vi "MacroAssert.vi"(8 "error in (no error)":errorcluster) -> (0 "error out":errorcluster)   [LabVIEW 2020, in "MacroAssert.lvlib"]
doc: "Presents an interface to create, edit, save, and execute user-defined macros."
uses:
  MacroAssert.lvlib
  Classes/Macro/Macro.lvclass
  Classes/Step/Step.lvclass
  <vilib>/Utility/miscctls.llb/LVRowAndColumnUnsignedTypeDef.ctl
  bd503c13-d10c-440e-ab5e-4e60baef5deb.vi
  SubVIs/FaKI State Machine/FaKI State Machine.lvlib
  CTLs/State Data.ctl
  CTLs/Hotkey Values.ctl
  CTLs/FGV Actions.ctl
  CTLs/Hotkey Type.ctl
  CTLs/Refs.ctl
  fa5aba67-e91f-4216-ac5c-c17457851557.vi
  CTLs/Report Data.ctl
  CTLs/Edit Action.ctl
  <vilib>/Utility/miscctls.llb/LVPositionTypeDef.ctl
  <vilib>/Utility/inputDevices.llb/closeKeyboard.vi
panel:
  in  "Report Path":path
  out "Status":string
  in  "Add Step 2":bool
  in  "Dbl Click":T1
  in  "Macro Steps":i32(listbox)
  out "Abort Hotkey":string
  out "Metadata":string
  in  "Description":string
  out "Resolutions":cluster{"Width":i16, "Height":i16}[](array[cluster])
  out "n Monitors":i32
  out "Macro Hotkey":string
  in  "Start/Stop":bool
  in  "N":i32 caption="Times to Repeat\n(-1 = indefinitely)" min=-1
  in  "Activation Type":enum32{"Hotkey", "Automatic"}(radio)
  out "Row":i32
  in  "Clear Steps":bool
  in  "Delete Step":bool
  in  "Insert Step":bool
  in  "Add Step":bool
  in  "Modify Step":bool
  in  "Macro Name":string(combo)
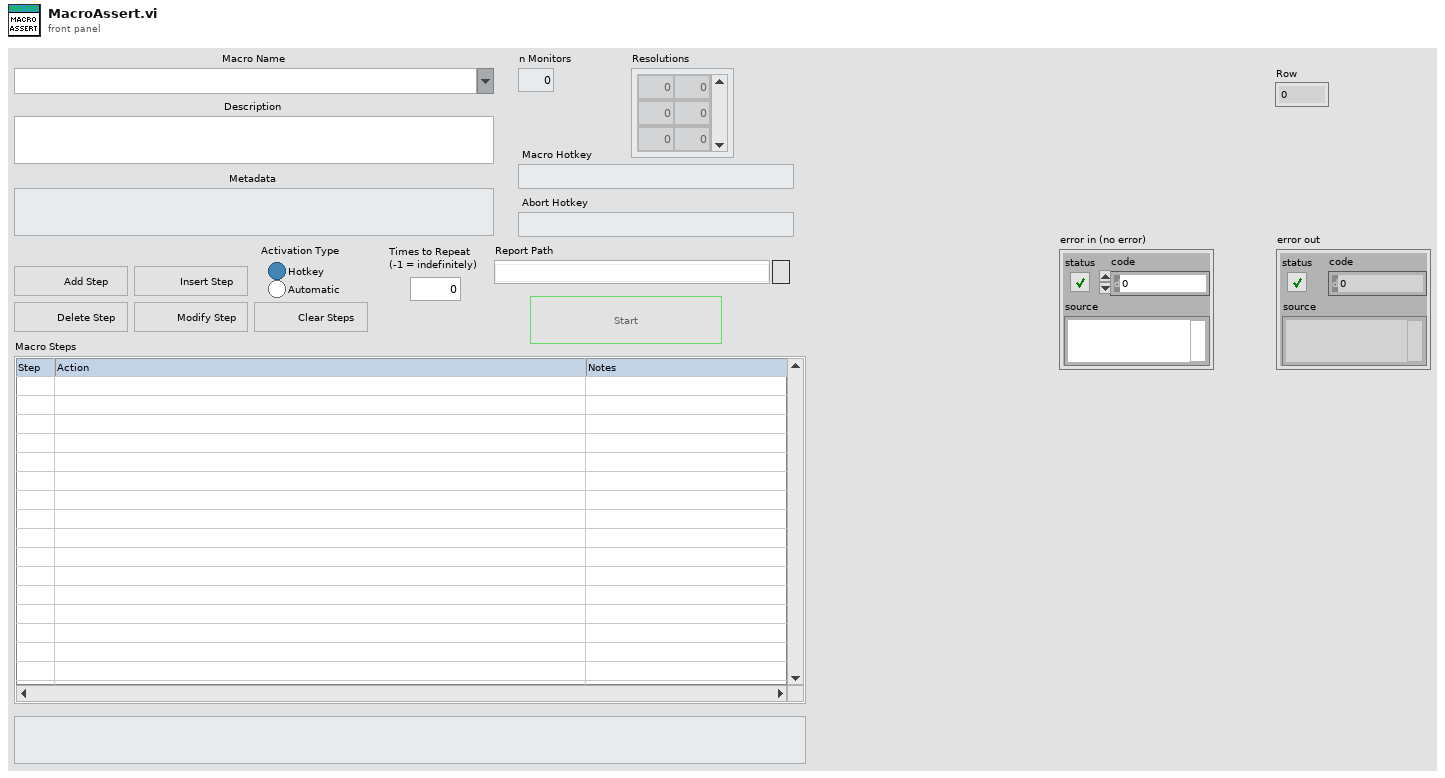
[diagram p1: front panel]
types:
  T1 = cluster{"Insert Before":bool, "Insert After":bool, "Modify Step 2":bool, "Delete Step 2":bool}
  T2 = typedef "LVPoint32TypeDef.ctl" = cluster{"Horizontal":i32, "Vertical":i32}
  T3 = enum32{"Invalid", "Standard", "Closed", "Hidden", "Minimized", "Maximized"}
  T4 = enum32{"invalid app kind", "Development System", "Run Time System", "Student Edition", "Embedded LabVIEW", "Evaluation", "Custom"}
  T5 = typedef "MacroAssert.lvlib/State Data.ctl" = cluster{"Core":cluster{"Current VI Reference":refnum<vi>, "Close Panel on Exit?":bool}, "Macro":cluster{"New":refnum<class "Macro.lvclass">, "Saved":refnum<class "Macro.lvclass">}, "Step":i32, "n":i32, "Hotkey Values":T6, "Keyboard":refnum<k1>, "Macro Active?":bool, "Macro Names":string[], "Rcount":i32, "Refs":T7, "Resolutions":cluster{"Width":i16, "Height":i16}[], "App Data Dir":path, "Start Time":timestamp, "Report Data":T8[]}
  T6 = typedef "MacroAssert.lvlib/Hotkey Values.ctl" = cluster{"Macro Hotkey":enum16{"0", "1", "2", "3", "4", "5", "6", "7", "8", "9", "A", "B", "C", "D", "E", "F", "G", "H", "I", "J", "K", "L", "M", "N", "O", "P", "Q", "R", "S", "T", "U", "V", "W", "X", "Y", "Z", "F1", "F2", "F3", "F4", "F5", "F6", "F7", "F8", "F9", "F10", "F11", "F12", "F13", "F14", "F15", "ADD", "BACK", "BACKSLASH", "CAPITAL", "COMMA", "DECIMAL", "DELETE", "DIVIDE", "DOWN", "END", "EQUALS", "ESCAPE", "GRAVE (`)", "HOME", "INSERT", "LBRACKET", "LCONTROL", "LEFT", "L ALT", "LSHIFT", "LWIN", "MINUS", "MULTIPLY", "NEXT", "NUMLOCK", "NUMPAD_0", "NUMPAD_1", "NUMPAD_2", "NUMPAD_3", "NUMPAD_4", "NUMPAD_5", "NUMPAD_6", "NUMPAD_7", "NUMPAD_8", "NUMPAD_9", "PAUSE", "PERIOD", "PRIOR (PG UP)", "RBRACKET", "RCONTROL", "RETURN", "RIGHT", "R ALT", "RSHIFT", "RWIN", "SCROLL", "SEMICOLON", "SLASH", "SPACE", "SUBTRACT", "TAB", "UP", "ENTER (num pad)", "' (quote)"}[], "Abort Hotkey":enum16{"0", "1", "2", "3", "4", "5", "6", "7", "8", "9", "A", "B", "C", "D", "E", "F", "G", "H", "I", "J", "K", "L", "M", "N", "O", "P", "Q", "R", "S", "T", "U", "V", "W", "X", "Y", "Z", "F1", "F2", "F3", "F4", "F5", "F6", "F7", "F8", "F9", "F10", "F11", "F12", "F13", "F14", "F15", "ADD", "BACK", "BACKSLASH", "CAPITAL", "COMMA", "DECIMAL", "DELETE", "DIVIDE", "DOWN", "END", "EQUALS", "ESCAPE", "GRAVE (`)", "HOME", "INSERT", "LBRACKET", "LCONTROL", "LEFT", "L ALT", "LSHIFT", "LWIN", "MINUS", "MULTIPLY", "NEXT", "NUMLOCK", "NUMPAD_0", "NUMPAD_1", "NUMPAD_2", "NUMPAD_3", "NUMPAD_4", "NUMPAD_5", "NUMPAD_6", "NUMPAD_7", "NUMPAD_8", "NUMPAD_9", "PAUSE", "PERIOD", "PRIOR (PG UP)", "RBRACKET", "RCONTROL", "RETURN", "RIGHT", "R ALT", "RSHIFT", "RWIN", "SCROLL", "SEMICOLON", "SLASH", "SPACE", "SUBTRACT", "TAB", "UP", "ENTER (num pad)", "' (quote)"}[]}
  T7 = typedef "MacroAssert.lvlib/Refs.ctl" = cluster{"Name":refnum<vi>, "Description":refnum<vi>, "Start":refnum<vi>, "Steps":refnum<vi>, "Simple Refs":refnum<vi>[]}
  T8 = typedef "MacroAssert.lvlib/Report Data.ctl" = cluster{"Step":string, "Pass?":bool, "Actual Value":variant}
  T9 = typedef "MacroAssert.lvlib/Edit Action.ctl" = enum16{"Add", "Insert", "Modify", "Delete", "Insert Before", "Insert After", "Modify 2", "Delete 2", "Clear All"}
  T10 = typedef "LVRowAndColumnUnsignedTypeDef.ctl" = cluster{"Row":u32, "Column":u32}
  T11 = enum8{"Enabled", "Disabled", "Disabled and Grayed Out"}
  T12 = typedef "LVPositionTypeDef.ctl" = cluster{"Left":i32, "Top":i32}
  T13 = typedef "MacroAssert.lvlib/Hotkey Type.ctl" = enum16{"Macro Hotkey", "Abort Hotkey"}
  T14 = typedef "MacroAssert.lvlib/FGV Actions.ctl" = enum16{"Read", "Write"}
  T15 = enum16{"0", "1", "2", "3", "4", "5", "6", "7", "8", "9", "A", "B", "C", "D", "E", "F", "G", "H", "I", "J", "K", "L", "M", "N", "O", "P", "Q", "R", "S", "T", "U", "V", "W", "X", "Y", "Z", "F1", "F2", "F3", "F4", "F5", "F6", "F7", "F8", "F9", "F10", "F11", "F12", "F13", "F14", "F15", "ADD", "BACK", "BACKSLASH", "CAPITAL", "COMMA", "DECIMAL", "DELETE", "DIVIDE", "DOWN", "END", "EQUALS", "ESCAPE", "GRAVE (`)", "HOME", "INSERT", "LBRACKET", "LCONTROL", "LEFT", "L ALT", "LSHIFT", "LWIN", "MINUS", "MULTIPLY", "NEXT", "NUMLOCK", "NUMPAD_0", "NUMPAD_1", "NUMPAD_2", "NUMPAD_3", "NUMPAD_4", "NUMPAD_5", "NUMPAD_6", "NUMPAD_7", "NUMPAD_8", "NUMPAD_9", "PAUSE", "PERIOD", "PRIOR (PG UP)", "RBRACKET", "RCONTROL", "RETURN", "RIGHT", "R ALT", "RSHIFT", "RWIN", "SCROLL", "SEMICOLON", "SLASH", "SPACE", "SUBTRACT", "TAB", "UP", "ENTER (num pad)", "' (quote)"}[]
  T16 = typedef "LVAllMonitorsDisplayTypeDef.ctl" = cluster{"Bounds":cluster{"Left":i16, "Top":i16, "Right":i16, "Bottom":i16}, "Depth":i16}[]
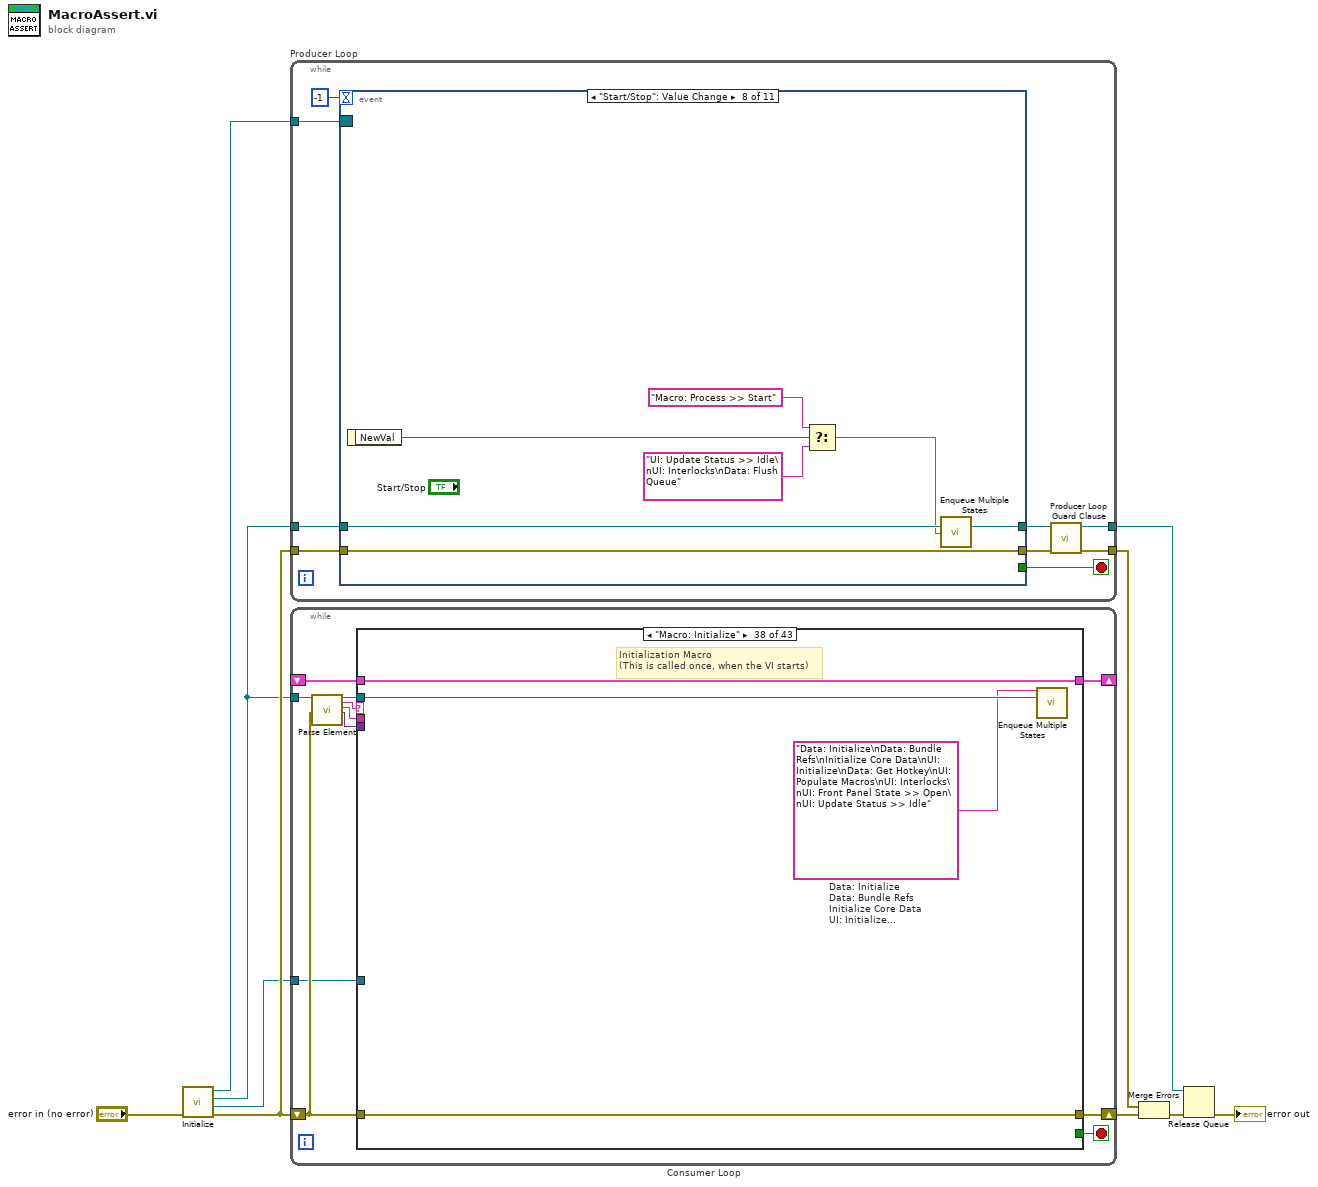
[diagram p0: block diagram]
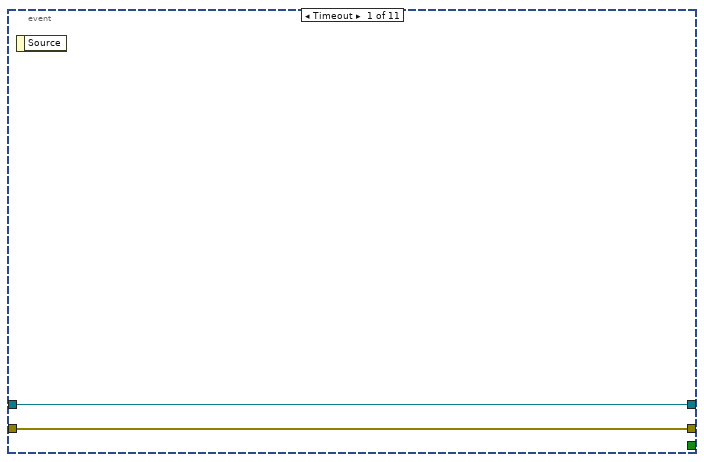
[diagram p2: hidden frame]
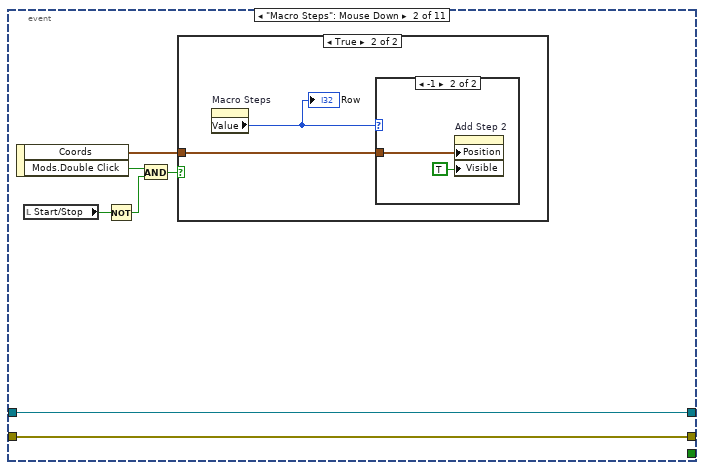
[diagram p3: hidden frame]
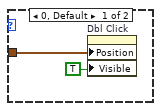
[diagram p5: hidden frame]
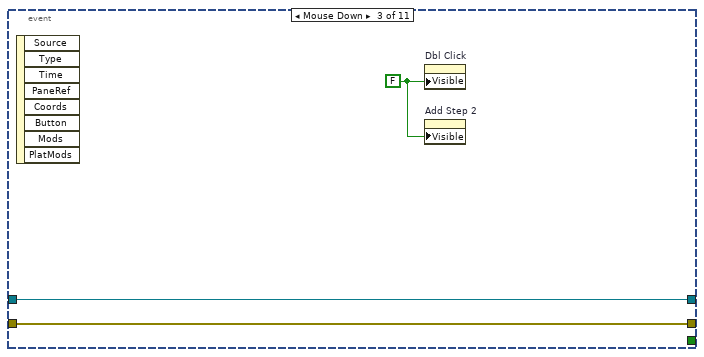
[diagram p6: hidden frame]
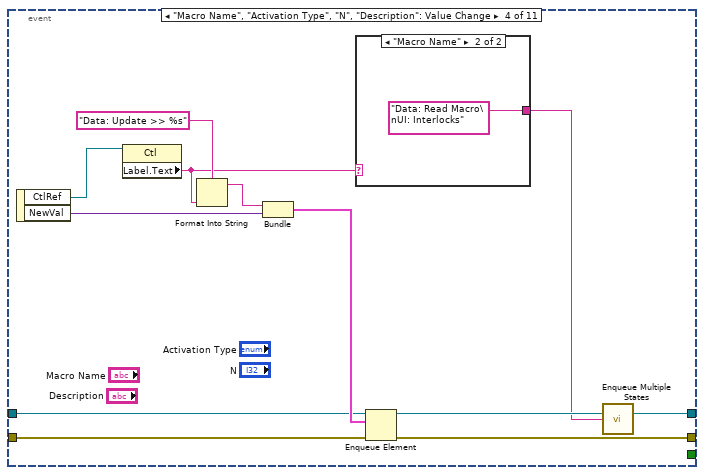
[diagram p7: hidden frame]
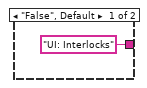
[diagram p8: hidden frame]
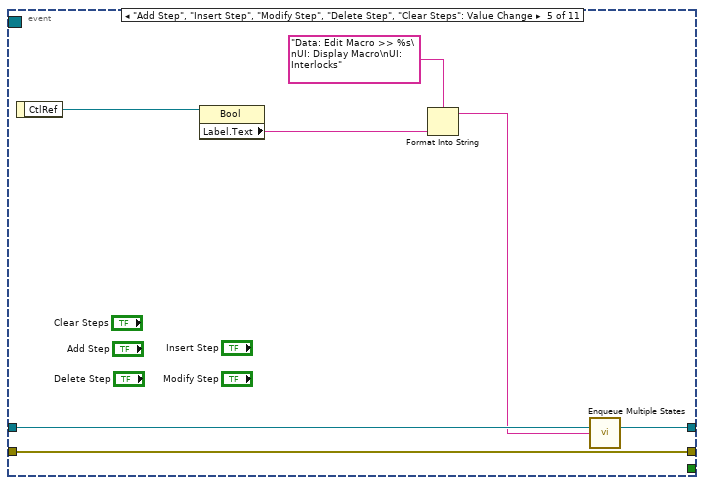
[diagram p9: hidden frame]
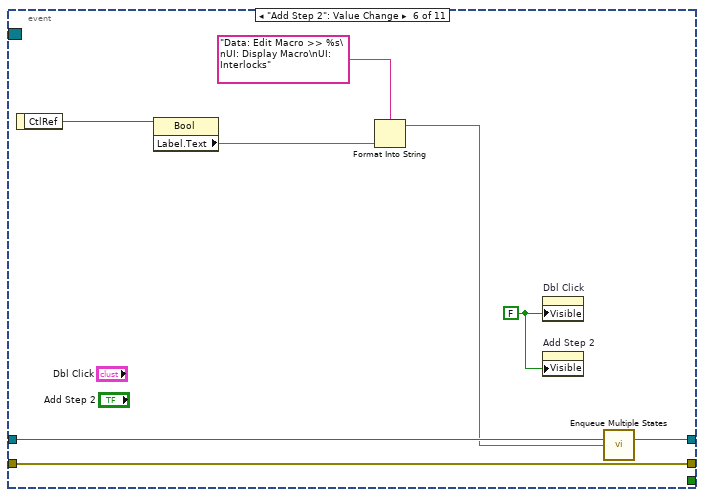
[diagram p10: hidden frame]
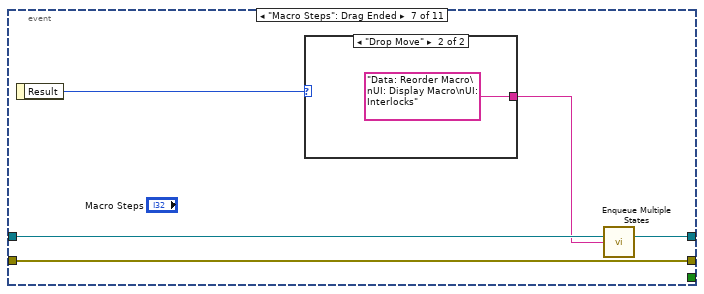
[diagram p11: hidden frame]
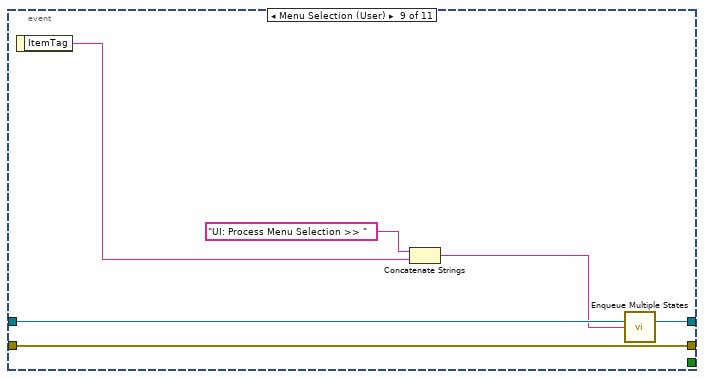
[diagram p13: hidden frame]
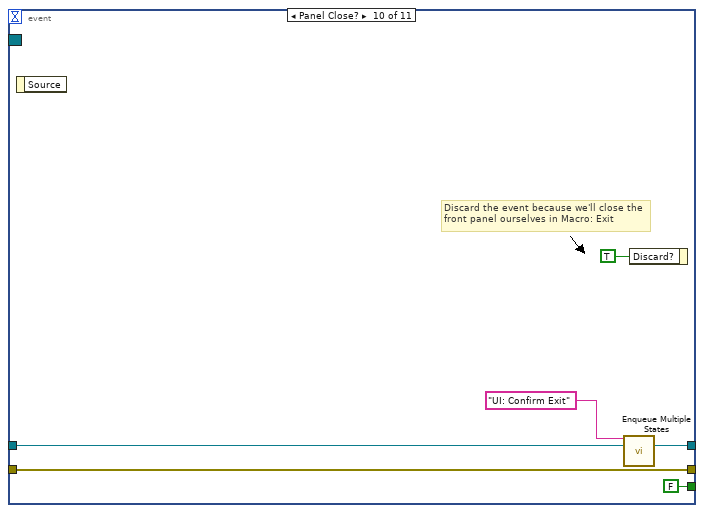
[diagram p14: hidden frame]
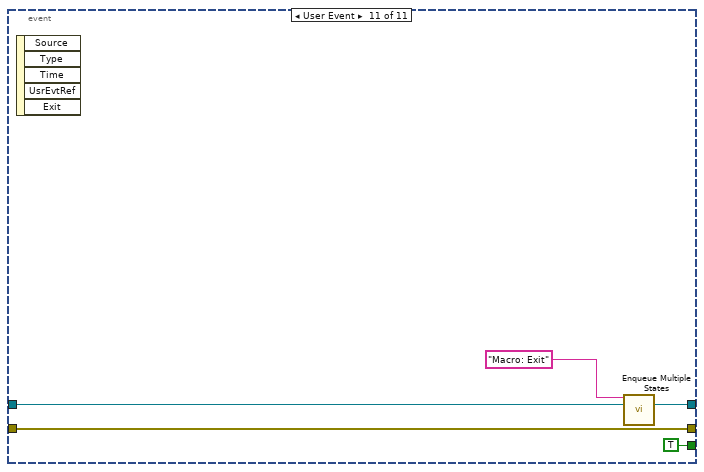
[diagram p15: hidden frame]
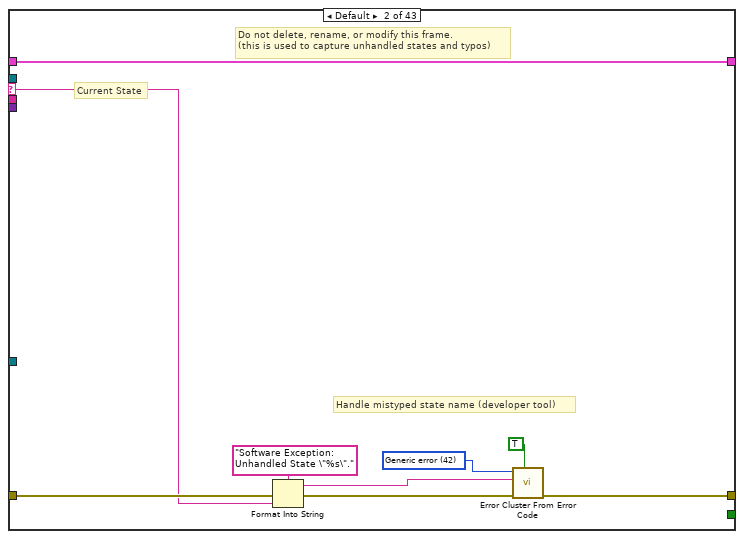
[diagram p17: hidden frame]
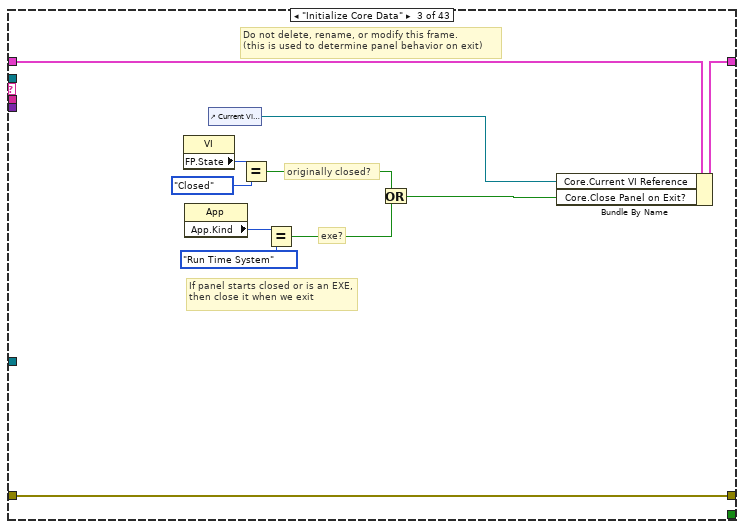
[diagram p18: hidden frame]
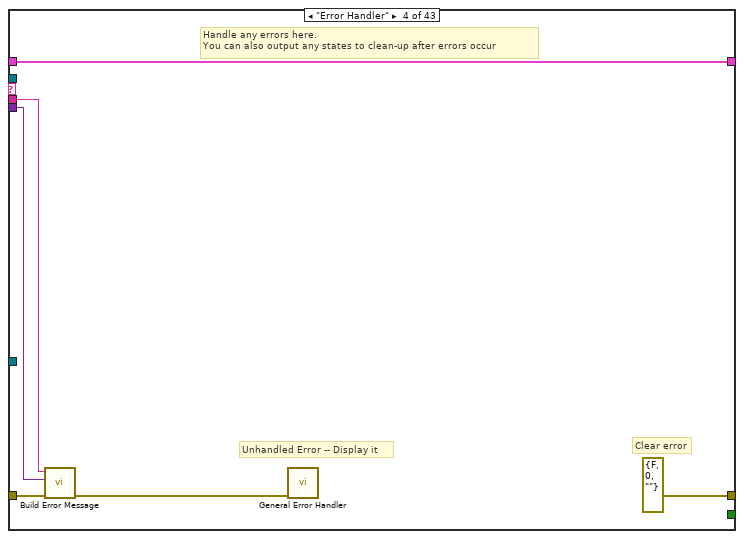
[diagram p19: hidden frame]
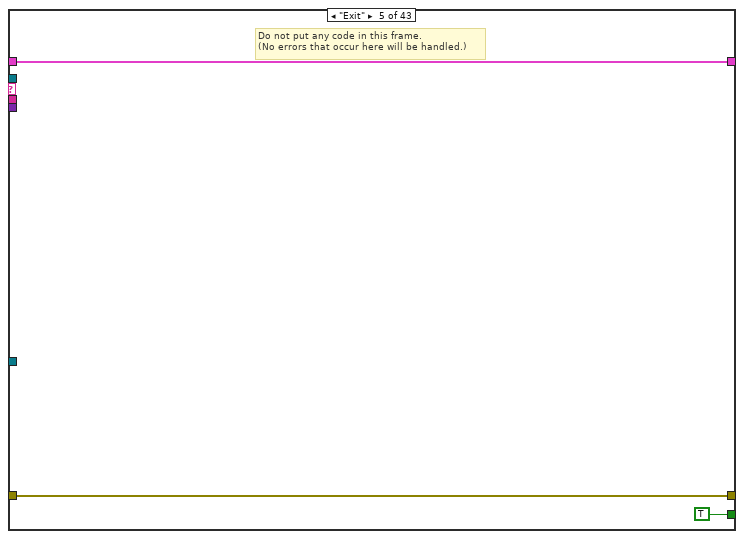
[diagram p20: hidden frame]
diagram:
  n1 = call "Initialize.vi"("error in (no error)"="error in (no error)") -> ("error out"=w5:errorcluster, "Exit Event"=w3:refnum<user-event>, "Queue"=w2:refnum<queue>, "Event Registration Refnum"=w1:refnum<event-registration>)  [unwired: 7 in]
  n2 = while "Producer Loop" {
    tunnel: w1 -> [w13]
    tunnel: w2 -> [w15]
    tunnel: [w18] -> w10
    tunnel: w5 -> [w17]
    tunnel: [w19] -> w8
    stop <- w12 stop-if-true
    n3 = event shown="[7] \"Start/Stop\": Value Change" {
      selector: w13 -> [_ _ _ _ _ _ _ _ _ _ _]
      dyn-events: _ -> [_ _ _ _ _ _ _ _ _ _ _]
      timeout: -1 ("Timeout") -> [_ _ _ _ _ _ _ _ _ _ _]
      tunnel: [w21 w28 w37 w45 w58 w66 w71 w79 w85 w91 w96] -> w16
      tunnel: w17 -> [w21 w28 w37 w48 w58 w66 w71 w79 w85 w91 w96]
      tunnel: w15 -> [w20 w26 w36 w38 w56 w63 w70 w75 w84 w88 w94]
      tunnel: [w20 w26 w36 w47 w55 w62 w69 w76 w83 w87 w93] -> w14
      tunnel: [_ _ _ _ _ _ _ _ _ FALSE TRUE] -> w12
      event Timeout {
        n4 = event-data() -> ()  [unwired: 1 in, 1 out]
      }
      event "Macro Steps": Mouse Down {
        n5 = event-data() -> ("Coords"=w27:T2, "Mods.Double Click"=w23:bool)  [unwired: 1 in]
        n6 = local read "Start/Stop"() -> (w25:bool)
        n7 = Not(x=w25) -> (.not. x?=w24:bool)
        n8 = And(x=w23, y=w24) -> (x .and. y?=w22:bool)
        n9 = case shown="True" w22 {
          tunnel: w27 -> [_ w30]
          frame False {
          }
          frame True {
            n10 = property on="Macro Steps" class="MCListbox (strict)"() -> ("Value"=w29:i32)  [unwired: 2 in, 2 out]
            "Row" <- w29
            n11 = case shown="-1" w29 {
              tunnel: w30 -> [w31 w33]
              frame 0, Default {
                n12 = property on="Dbl Click" class="Clust"("Position"=w31, "Visible"=TRUE) -> ()  [unwired: 2 in, 2 out]
              }
              frame -1 {
                n13 = property on="Add Step 2" class="Bool"("Position"=w33, "Visible"=TRUE) -> ()  [unwired: 2 in, 2 out]
              }
            }
          }
        }
      }
      event Mouse Down {
        w35 = FALSE ("Visible")
        n14 = event-data() -> ()  [unwired: 1 in, 8 out]
        n15 = property on="Dbl Click" class="Clust"("Visible"=w35) -> ()  [unwired: 2 in, 2 out]
        n16 = property on="Add Step 2" class="Bool"("Visible"=w35) -> ()  [unwired: 2 in, 2 out]
      }
      event "Macro Name", "Activation Type", "N", "Description": Value Change {
        n17 = event-data() -> ("CtlRef"=w44:refnum<vi>, "NewVal"=w41:variant)  [unwired: 1 in]
        n18 = property class="Ctl"(reference=w44) -> ("Label.Text"=w40:string)  [unwired: 1 in, 2 out]
        n19 = Format Into String(format string="Data: Update >> %s", w40) -> (resulting string=w42:string)  [unwired: 2 in, 1 out]
        n20 = Bundle(w42, "NewVal"=w41) -> (w39:cluster{string, "NewVal":variant})  [unwired: 1 in]
        n21 = case shown="\"Macro Name\"" w40 {
          tunnel: ["UI: Interlocks" ("string") "Data: Read Macro\nUI: Interlocks" ("string")] -> w46
          frame "False", Default {
          }
          frame "Macro Name" {
          }
        }
        n22 = Enqueue Element(queue=w38, element=w39, error in (no error)=w48) -> (queue out=w49:refnum<queue>, error out=w45:errorcluster)  [unwired: 1 in, 1 out]
        n23 = call "Enqueue Multiple States.vi"("queue in"=w49, "State(s) at Back"=w46) -> ("queue out"=w47:refnum<queue>)  [unwired: 13 in]
      }
      event "Add Step", "Insert Step", "Modify Step", "Delete Step", "Clear Steps": Value Change {
        n24 = event-data() -> ("CtlRef"=w57:refnum<vi>)  [unwired: 1 in]
        n25 = property class="Bool"(reference=w57) -> ("Label.Text"=w54:string)  [unwired: 1 in, 2 out]
        n26 = Format Into String(format string="Data: Edit Macro >> %s\nUI: Display Macro\nUI: Interlocks", w54) -> (resulting string=w52:string)  [unwired: 2 in, 1 out]
        n27 = call "Enqueue Multiple States.vi"("queue in"=w56, "State(s) at Back"=w52) -> ("queue out"=w55:refnum<queue>)  [unwired: 13 in]
      }
      event "Dbl Click.Insert Before", "Dbl Click.Insert After", "Dbl Click.Modify Step 2", "Dbl Click.Delete Step 2", "Add Step 2": Value Change {
        w64 = FALSE ("Visible")
        n28 = event-data() -> ("CtlRef"=w65:refnum<vi>)  [unwired: 1 in]
        n29 = property class="Bool"(reference=w65) -> ("Label.Text"=w60:string)  [unwired: 1 in, 2 out]
        n30 = Format Into String(format string="Data: Edit Macro >> %s\nUI: Display Macro\nUI: Interlocks", w60) -> (resulting string=w59:string)  [unwired: 2 in, 1 out]
        n31 = property on="Dbl Click" class="Clust"("Visible"=w64) -> ()  [unwired: 2 in, 2 out]
        n32 = property on="Add Step 2" class="Bool"("Visible"=w64) -> ()  [unwired: 2 in, 2 out]
        n33 = call "Enqueue Multiple States.vi"("queue in"=w63, "State(s) at Back"=w59) -> ("queue out"=w62:refnum<queue>)  [unwired: 13 in]
      }
      event "Macro Steps": Drag Ended {
        n34 = event-data() -> ("Result"=w67:enum16{"Drop Cancel", "Drop Move", "Drop Copy"})  [unwired: 1 in]
        n35 = case shown="\"Drop Move\"" w67 {
          tunnel: [_ "Data: Reorder Macro\nUI: Display Macro\nUI: Interlocks" ("State(s) at Back")] -> w68
          frame "Drop Cancel", Default {
          }
          frame "Drop Move" {
          }
        }
        n36 = call "Enqueue Multiple States.vi"("queue in"=w70, "State(s) at Back"=w68) -> ("queue out"=w69:refnum<queue>)  [unwired: 13 in]
      }
      event "Start/Stop": Value Change {
        n37 = event-data() -> ("NewVal"=w78:bool)  [unwired: 1 in]
        n38 = Select(t="Macro: Process >> Start", s=w78, f="UI: Update Status >> Idle\nUI: Interlocks\nData: Flush Queue") -> (s? t:f=w74:string)
        n39 = call "Enqueue Multiple States.vi"("queue in"=w75, "State(s) at Back"=w74) -> ("queue out"=w76:refnum<queue>)  [unwired: 13 in]
      }
      event Menu Selection (User) {
        n40 = event-data() -> ("ItemTag"=w81:string)  [unwired: 1 in]
        n41 = Concatenate Strings("UI: Process Menu Selection >> ", w81) -> (w80:string)
        n42 = call "Enqueue Multiple States.vi"("queue in"=w84, "State(s) at Back"=w80) -> ("queue out"=w83:refnum<queue>)  [unwired: 13 in]
      }
      event Panel Close? {
        # "Discard the event because we'll close the front panel ourselves in Macro: Exit"
        n43 = event-data() -> ()  [unwired: 1 in, 1 out]
        n44 = call "Enqueue Multiple States.vi"("State(s) at Front"="UI: Confirm Exit", "queue in"=w88) -> ("queue out"=w87:refnum<queue>)  [unwired: 13 in]
        n45 = event-data("Discard?"=TRUE) -> ()  [unwired: 1 in, 1 out]
      }
      event User Event {
        n46 = event-data() -> ()  [unwired: 1 in, 5 out]
        n47 = call "Enqueue Multiple States.vi"("State(s) at Front"="Macro: Exit", "queue in"=w94) -> ("queue out"=w93:refnum<queue>)  [unwired: 13 in]
      }
    }
    n48 = call "Producer Loop Guard Clause.vi"("error in (no error)"=w16, "queue in"=w14) -> ("error out"=w19:errorcluster, "queue out"=w18:refnum<queue>)  [unwired: 8 in]
  }
  n49 = while "Consumer Loop" {
    shift-right: [w98] -> _
    shift-left: _ -> [w103]
    shift-right: [w105] -> w7
    shift-left: w5 -> [w106]
    tunnel: w2 -> [w107]
    tunnel: w3 -> [w97]
    stop <- w104 stop-if-true
    n50 = call "Parse Element.vi"("queue in"=w107, "error in (no error)"=w106) -> ("queue out"=w102:refnum<queue>, "State"=w101:string, "Arg"=w100:string, "Data"=w99:variant)  [unwired: 14 in]
    n51 = case shown="\"Macro: Initialize\"" w101 {
      selector: w101 -> [_ w110 _ _ _ _ _ _ _ _ _ _ _ _ _ _ _ _ _ _ _ _ _ _ _ _ _ _ _ _ _ _ _ _ _ _ _ _ _ _ _ _ _]
      tunnel: w102 -> [_ _ _ _ _ _ _ _ _ _ _ _ _ _ _ _ w337 w358 _ _ _ _ _ _ _ w478 _ _ _ w547 w562 _ _ w583 w592 _ _ w627 w631 w632 w709 _ w725]
      tunnel: w100 -> [_ _ _ w131 _ _ _ _ w168 _ _ _ w253 _ _ _ _ _ _ _ _ _ w393 w401 _ w479 _ _ w501 _ _ _ _ _ _ _ _ _ _ w636 _ _ _]
      tunnel: w103 -> [w108 w112 w124 w134 w138 w139 _ w154 w169 w223 w237 w243 w254 w303 w315 w327 w333 w359 w367 w368 w372 w390 w396 w403 w475 w483 w487 w499 w502 w546 w565 w573 w576 w582 w593 w616 w622 w625 w629 w633 w713 w715 w724]
      tunnel: [w109 w114 w128 errorcluster {"status"=FALSE, "code"=0, "source"=""} ("error out") w137 w140 w142 w155 w164 w224 w235 w244 w256 w304 w320 w328 w335 w360 w365 w369 w375 w391 w394 w404 w476 w481 w489 w497 w503 w540 w561 w571 w574 w580 w589 w610 w623 w626 w630 w637 w714 w716 w721] -> w105
      tunnel: w106 -> [w109 w113 w128 w133 w137 w140 w147 w155 w167 w224 w229 w245 w256 w304 w320 w329 w336 w360 w364 w369 w375 w391 w395 w405 w476 w482 w490 w497 w503 w549 w566 w572 w575 w580 w589 w614 w623 w626 w630 w637 w714 w716 w722]
      tunnel: [_ _ _ _ TRUE _ _ _ _ _ _ _ _ _ _ _ _ _ _ _ _ _ _ _ _ _ _ _ _ _ _ _ _ _ _ _ _ _ _ _ _ _ _] -> w104
      tunnel: w99 -> [_ _ _ w130 _ _ _ _ w166 _ _ _ _ _ _ _ _ _ _ _ _ _ _ _ _ _ _ _ _ _ _ _ _ _ _ _ _ _ _ _ _ _ _]
      tunnel: [w108 w112 w129 w134 w138 w139 w143 w153 w165 w222 w236 w243 w255 w302 w314 w326 w334 w359 w367 w368 w370 w390 w396 w403 w475 w483 w488 w499 w502 w546 w565 w573 w576 w582 w591 w616 w622 w625 w629 w635 w713 w715 w723] -> w98
      tunnel: w97 -> [_ _ _ _ _ _ _ _ _ _ _ _ _ _ _ _ _ _ _ _ _ _ _ _ _ _ _ _ _ _ _ _ _ _ _ w608 _ _ _ _ _ _ _]
      frame "---------- Core ----------" {
        # "Do not put any code in this frame.\n(it is a separator no-op)"
      }
      frame Default {
        w117 = 42 items=["No error", "Argument error", "Memory is full", "Out of zone", "End of file", "File already open", "Generic file I/O error", "File not found", "File permission error", "Disk is full", "Duplicate path", "Too many files open", "System feature not enabled", "Resource file not found", "Cannot add resource", "Resource not found", "Image not found", "Image memory error", "Pen does not exist", "Config type invalid", "Config token not found", "Config parse error", "Config memory error", "Bad external code format", "Bad external code offset", "External code not present", "Null window", "Destroy window error", "Null menu", "Print aborted", "Bad print record", "Print driver error", "Windows error during printing", "Memory error during printing", "Print dialog error", "Generic print error", "Invalid device refnum", "Device not found", "Device parameter error", "Device unit error", "Cannot open device", "Device call aborted", "Generic error", "Cancelled by user", "Object ID too low", "Object ID too high", "Object not in heap", "Unknown heap", "Unknown object (invalid DefProc)", "Unknown object (DefProc not in table)", "Message out of range", "Invalid (null) method", "Unknown message", "Manager call not supported", "Bad address", "Network operation in progress", "Network operation timed out", "Connection is busy", "Network attribute not supported", "Network error", "Address in use", "System out of memory", "Connection aborted", "Connection refused", "Not connected", "Already connected", "Connection closed", "Initialization error (interapplication manager)", "Bad occurrence", "Wait on unbound occurrence handler", "Occurrence queue overflow", "Datalog type conflict", "Unused", "Unrecognized type (interapplication manager)", "Memory corrupt", "Failed to make temporary DLL", "Old CIN version", "Drag socket not found", "Failed to load drop-object", "Failed to register OLE object", "Failed to release OLE object", "Format specifier type mismatch", "Unknown format specifier", "Too few format specifiers", "Too many format specifiers", "Scan failed", "Newer CIN version", "Error converting to variant", "Runtime menu error", "Password tampered", "Variant attribute not found", "Incompatible variant data type", "Event data is not available", "Event Store is not present", "Occurrence is not found", "Event Queue is not created", "Event info is not available", "Refnum passed is NULL", "Error retrieving Class GUID", "Error retrieving CoClass GUID", "Error retrieving TypeLib GUID.", "Bad built application magic bytes.", "Specific driver is different from the specific driver associated with the Logical Name.", "There is no session opened to the class driver.", "Max Error", "MAX - Error with config objects", "MAX - Error loading configuration", "MAX - Group not supported"]
        # "Current State"
        # "Do not delete, rename, or modify this frame.\n(this is used to capture unhandled states and typos)"
        # "Handle mistyped state name (developer tool)"
        n52 = Format Into String(format string="Software Exception: Unhandled State \"%s\"." ("message"), error in=w113, w110) -> (resulting string=w116:string, error out=w115:errorcluster)  [unwired: 1 in]
        n53 = call <vilib>:"Error Cluster From Error Code.vi"("show call chain? (False)"=TRUE, "error in (no error)"=w115, "error message (\"\")"=w116, "error code (0)"=w117) -> ("error out"=w114:errorcluster)  [unwired: 5 in]
      }
      frame "Initialize Core Data" {
        # "Do not delete, rename, or modify this frame.\n(this is used to determine panel behavior on exit)"
        # "originally closed?"
        # "exe?"
        # "If panel starts closed or is an EXE, then close it when we exit"
        n54 = property class="VI"() -> ("FP.State"=w121:T3)  [unwired: 2 in, 2 out]
        n55 = property class="App"() -> ("App.Kind"=w127:T4)  [unwired: 2 in, 2 out]
        n56 = control-ref of="Current VI Reference"() -> (w122:refnum<vi>)
        n57 = Equal?(x=w121, y=T3."Closed" ("Front Panel Window:State")) -> (x = y?=w119:bool)
        n58 = Equal?(x=w127, y=T4."Run Time System" ("Application:Kind")) -> (x = y?=w125:bool)
        n59 = Or(x=w119, y=w125) -> (x .or. y?=w123:bool)
        n60 = Bundle By Name(cluster=w124, "Core.Current VI Reference"=w122, "Core.Close Panel on Exit?"=w123) -> (w129:T5)
      }
      frame "Error Handler" {
        # "Unhandled Error -- Display it"
        # "Handle any errors here.\nYou can also output any states to clean-up after errors occur"
        # "Clear error"
        n61 = call "Build Error Message.vi"("error in (no error)"=w133, "Data"=w130, "Arg"=w131) -> ("error out"=w132:errorcluster)  [unwired: 8 in]
        n62 = call <vilib>:"General Error Handler.vi"("error in (no error)"=w132) -> ()  [unwired: 10 in, 5 out]
      }
      frame "Exit" {
        # "Do not put any code in this frame.\n(No errors that occur here will be handled.)"
      }
      frame "---------- Data ----------" {
        # "Do not put any code in this frame.\n(It is a separator no-op. You can make a copy of this frame to create a new Data frame)"
      }
      frame "Data: Initialize" {
        # "Initialize the shift-register data, here."
        n63 = call <vilib>:"Intialize Keyboard.vi"("error in (no error)"=w147) -> ("error out"=w146:errorcluster, "device ID"=w144:refnum<k1>)  [unwired: 9 in]
        n64 = call "App Data Directory.vi"("error in (no error)"=w146) -> ("error out"=w142:errorcluster, "App Data Directory"=w141:path)  [unwired: 9 in]
        n65 = Bundle By Name(cluster=T5 {"Core"={"Current VI Reference"=refnum, "Close Panel on Exit?"=FALSE}, "Macro"={"New"=refnum, "Saved"=refnum}, "Step"=0, "n"=0, "Hotkey Values"={"Macro Hotkey"=[], "Abort Hotkey"=[]}, "Keyboard"=refnum, "Macro Active?"=FALSE, "Macro Names"=[], "Rcount"=0, "Refs"={"Name"=refnum, "Description"=refnum, "Start"=refnum, "Steps"=refnum, "Simple Refs"=[]}, "Resolutions"=[], "App Data Dir"=path "", "Start Time"=timestamp(0 s since 1904-01-01), "Report Data"=[]}, "Keyboard"=w144, "App Data Dir"=w141) -> (w143:T5)
      }
      frame "Data: Bundle Refs" {
        n66 = control-ref of="Activation Type"() -> (w158:refnum<vi>)
        n67 = control-ref of="Macro Name"() -> (w156:refnum<vi>)
        n68 = control-ref of="Add Step"() -> (w163:refnum<vi>)
        n69 = control-ref of="Delete Step"() -> (w161:refnum<vi>)
        n70 = control-ref of="Insert Step"() -> (w160:refnum<vi>)
        n71 = control-ref of="Modify Step"() -> (w162:refnum<vi>)
        n72 = control-ref of="Clear Steps"() -> (w159:refnum<vi>)
        n73 = control-ref of="N"() -> (w157:refnum<vi>)
        n74 = control-ref of="Macro Steps"() -> (w148:refnum<vi>)
        n75 = control-ref of="Macro Name"() -> (w152:refnum<vi>)
        n76 = control-ref of="Start/Stop"() -> (w150:refnum<vi>)
        n77 = control-ref of="Description"() -> (w151:refnum<vi>)
        n78 = Build Array(w163, w161, w160, w162, w159, w158, w157, w156) -> (w149:refnum<vi>[])
        n79 = Bundle By Name(cluster=w154, "Refs.Name"=w152, "Refs.Description"=w151, "Refs.Start"=w150, "Refs.Steps"=w148, "Refs.Simple Refs"=w149) -> (w153:T5)
      }
      frame "Data: Update" {
        n80 = case shown="\"Macro Name\"" w168 {
          selector: w168 -> [w170 _ _ _ _ _]
          tunnel: w169 -> [w173 w177 w187 w197 w206 w218]
          tunnel: w167 -> [w174 w181 w191 w201 w211 w221]
          tunnel: w166 -> [_ w180 w190 w200 w210 w220]
          tunnel: [w173 w176 w186 w196 w207 w217] -> w165
          tunnel: [w172 w178 w189 w199 w209 w216] -> w164
          frame Default {
            n81 = call "Unhandled String Argument--error.vi"("Argument"=w170) -> ("error out"=w171:errorcluster)  [unwired: 10 in]
            n82 = Merge Errors(w174, w171) -> (w172:errorcluster)
          }
          frame "Macro Name" {
            n83 = Variant To Data(error in=w181, type="", Variant=w180) -> (data=w175:string, error out=w178:errorcluster)
            n84 = in-place {
              in-place-border: w175 -> [w182]
              n85 = in-place-cluster #1(w177) -> ("Macro.New"=w184:refnum<class "Macro.lvclass">)
              n86 = property class="Macro.lvclass"(reference=w184, "Accessors:Name"=w182) -> (reference out=w183:refnum<class "Macro.lvclass">)  [unwired: 1 in, 1 out]
              n87 = in-place-cluster #1("Macro.New"=w183) -> (w176:T5)
            }
          }
          frame "Activation Type" {
            n88 = Variant To Data(error in=w191, type=enum32{"Hotkey", "Automatic"}."Hotkey" ("FP CTLs.Type"), Variant=w190) -> (data=w185:enum32{"Hotkey", "Automatic"}, error out=w189:errorcluster)
            n89 = in-place {
              in-place-border: w185 -> [w192]
              n90 = in-place-cluster #2(w187) -> ("Macro.New"=w194:refnum<class "Macro.lvclass">)
              n91 = property class="Macro.lvclass"(reference=w194, "Accessors:Activation Type"=w192) -> (reference out=w193:refnum<class "Macro.lvclass">)  [unwired: 1 in, 1 out]
              n92 = in-place-cluster #2("Macro.New"=w193) -> (w186:T5)
            }
          }
          frame "N" {
            n93 = Variant To Data(error in=w201, type=0 ("FP CTLs.N"), Variant=w200) -> (data=w195:i32, error out=w199:errorcluster)
            n94 = in-place {
              in-place-border: w195 -> [w202]
              n95 = in-place-cluster #3(w197) -> ("Macro.New"=w204:refnum<class "Macro.lvclass">)
              n96 = property class="Macro.lvclass"(reference=w204, "Accessors:N"=w202) -> (reference out=w203:refnum<class "Macro.lvclass">)  [unwired: 1 in, 1 out]
              n97 = in-place-cluster #3("Macro.New"=w203) -> (w196:T5)
            }
          }
          frame "Description" {
            n98 = Variant To Data(error in=w211, type="" ("FP CTLs.N"), Variant=w210) -> (data=w205:string, error out=w209:errorcluster)
            n99 = in-place {
              in-place-border: w205 -> [w212]
              n100 = in-place-cluster #4(w206) -> ("Macro.New"=w214:refnum<class "Macro.lvclass">)
              n101 = property class="Macro.lvclass"(reference=w214, "Accessors:Description"=w212) -> (reference out=w213:refnum<class "Macro.lvclass">)  [unwired: 1 in, 1 out]
              n102 = in-place-cluster #4("Macro.New"=w213) -> (w207:T5)
            }
          }
          frame "Macro Active?" {
            n103 = Variant To Data(error in=w221, type=FALSE, Variant=w220) -> (data=w219:bool, error out=w216:errorcluster)
            n104 = Bundle By Name(cluster=w218, "Macro Active?"=w219) -> (w217:T5)
          }
        }
      }
      frame "Data: Increment Step" {
        n105 = in-place {
          n106 = in-place-cluster #5(w223) -> ("Step"=w226:i32)
          n107 = Increment(x=w226) -> (x+1=w225:i32)
          n108 = in-place-cluster #5("Step"=w225) -> (w222:T5)
        }
      }
      frame "Data: Get Hotkey" {
        n109 = call "App Config INI.vi"("error in (no error)"=w229) -> ("error out"=w228:errorcluster, "App Config"=w227:path)  [unwired: 9 in]
        n110 = call "Get Hotkey.vi"("error in (no error)"=w228, "File Path"=w227) -> ("error out"=w235:errorcluster, "Hotkey Values"=w233:T6)  [unwired: 8 in]
        n111 = Unbundle By Name(w233) -> ("Macro Hotkey"=w232:T15, "Abort Hotkey"=w230:T15)
        n112 = Bundle By Name(cluster=w237, "Hotkey Values"=w233) -> (w236:T5)
        n113 = call "Convert Hotkey to String.vi"("Hotkey"=w232) -> ("String"=→"Macro Hotkey":string)  [unwired: 10 in]
        n114 = call "Convert Hotkey to String.vi"("Hotkey"=w230) -> ("String"=→"Abort Hotkey":string)  [unwired: 10 in]
      }
      frame "Data: Build Report" {
        n115 = Unbundle By Name(w243) -> ("Macro.New"=w242:refnum<class "Macro.lvclass">, "Report Data"=w241:T8[])
        n116 = Empty String/Path?(string/path="Report Path") -> (empty?=w239:bool)
        n117 = Not(x=w239) -> (.not. x?=w238:bool)
        n118 = case shown="True" w238 {
          tunnel: w245 -> [w246 w251]
          tunnel: [w246 w250] -> w244
          tunnel: w242 -> [_ w249]
          tunnel: w241 -> [_ w248]
          tunnel: "Report Path" -> [_ w247]
          frame False {
          }
          frame True {
            n119 = call-dynamic "Build Report.vi"("error in (no error)"=w251, "Report Data"=w248, "Path"=w247, "Macro in"=w249) -> ("error out"=w250:errorcluster)  [unwired: 6 in, 1 out]
          }
        }
      }
      frame "Data: Edit Macro" {
        n120 = local read "Row"() -> (w252:i32)
        n121 = in-place {
          in-place-border: w253 -> [w258]
          in-place-border: w252 -> [w257]
          n122 = in-place-cluster #6(w254) -> ("Macro.New"=w260:refnum<class "Macro.lvclass">)
          n123 = case shown="\"Add Step\"" w258 {
            tunnel: w260 -> [w261 w263 w266 w269 w272 w276 w278 w282 w287 w291 w295]
            tunnel: [w261 w262 w265 w268 w271 w275 w277 w281 w286 w290 w294] -> w259
            tunnel: w257 -> [_ _ _ _ _ _ w279 w284 w288 w292 _]
            frame Default {
            }
            frame "Add Step" {
              n124 = call-dynamic "Edit.vi"("Action"=Edit_Action."Add", "Macro in"=w263) -> ("Macro out"=w262:refnum<class "Macro.lvclass">)  [unwired: 8 in, 1 out]
            }
            frame "Insert Step" {
              n125 = call-dynamic "Edit.vi"("Action"=Edit_Action."Insert", "Macro in"=w266) -> ("Macro out"=w265:refnum<class "Macro.lvclass">)  [unwired: 8 in, 1 out]
            }
            frame "Modify Step" {
              n126 = call-dynamic "Edit.vi"("Action"=Edit_Action."Modify", "Macro in"=w269) -> ("Macro out"=w268:refnum<class "Macro.lvclass">)  [unwired: 8 in, 1 out]
            }
            frame "Delete Step" {
              n127 = call-dynamic "Edit.vi"("Action"=Edit_Action."Delete", "Macro in"=w272) -> ("Macro out"=w271:refnum<class "Macro.lvclass">)  [unwired: 8 in, 1 out]
            }
            frame "Add Step 2" {
              n128 = call-dynamic "Edit.vi"("Action"=Edit_Action."Add", "Macro in"=w276) -> ("Macro out"=w275:refnum<class "Macro.lvclass">)  [unwired: 8 in, 1 out]
            }
            frame "Insert Before" {
              n129 = call-dynamic "Edit.vi"("Action"=Edit_Action."Insert Before", "Step"=w279, "Macro in"=w278) -> ("Macro out"=w277:refnum<class "Macro.lvclass">)  [unwired: 7 in, 1 out]
            }
            frame "Insert After" {
              n130 = Increment(x=w284) -> (x+1=w283:i32)
              n131 = call-dynamic "Edit.vi"("Action"=Edit_Action."Insert After", "Step"=w283, "Macro in"=w282) -> ("Macro out"=w281:refnum<class "Macro.lvclass">)  [unwired: 7 in, 1 out]
            }
            frame "Modify Step 2" {
              n132 = call-dynamic "Edit.vi"("Action"=Edit_Action."Modify 2", "Step"=w288, "Macro in"=w287) -> ("Macro out"=w286:refnum<class "Macro.lvclass">)  [unwired: 7 in, 1 out]
            }
            frame "Delete Step 2" {
              n133 = call-dynamic "Edit.vi"("Action"=Edit_Action."Delete 2", "Step"=w292, "Macro in"=w291) -> ("Macro out"=w290:refnum<class "Macro.lvclass">)  [unwired: 7 in, 1 out]
            }
            frame "Clear Steps" {
              n134 = call "Confirm Clear"() -> ("OK"=w296:bool)  [unwired: 10 in, 1 out]
              n135 = case shown="True" w296 {
                tunnel: w295 -> [w297 w300]
                tunnel: [w297 w299] -> w294
                frame False {
                }
                frame True {
                  n136 = property on="Macro Steps" class="MCListbox (strict)"("TopLeft"=T10 {"Row"=0, "Column"=0} ("Index Values")) -> ()  [unwired: 2 in, 2 out]
                  n137 = call-dynamic "Edit.vi"("Action"=Edit_Action."Clear All", "Macro in"=w300) -> ("Macro out"=w299:refnum<class "Macro.lvclass">)  [unwired: 8 in, 1 out]
                }
              }
            }
          }
          n138 = in-place-cluster #6("Macro.New"=w259) -> (w255:T5)
        }
      }
      frame "Data: Bundle Macro" {
        n139 = in-place {
          n140 = in-place-cluster #7(w303) -> ("Resolutions"=w309:cluster{"Width":i16, "Height":i16}[], "Macro.New"=w312:refnum<class "Macro.lvclass">)
          n141 = property class="Macro.lvclass"(reference=w312) -> (reference out=w310:refnum<class "Macro.lvclass">, "Accessors:Date Created"=w307:timestamp)  [unwired: 1 in, 1 out]
          n142 = Get Date/Time In Seconds() -> (seconds since 1Jan1904=w305:timestamp)
          n143 = Not Equal To 0?(x=w307) -> (x != 0?=w308:bool)
          n144 = Select(t=w307, s=w308, f=w305) -> (s? t:f=w306:timestamp)
          n145 = property class="Macro.lvclass"(reference=w310, "Accessors:Resolutions"=w309, "Accessors:Date Created"=w306, "Accessors:Date Updated"=w305) -> (reference out=w311:refnum<class "Macro.lvclass">)  [unwired: 1 in, 1 out]
          n146 = in-place-cluster #7("Resolutions"=w309, "Macro.New"=w311) -> (w302:T5)
        }
      }
      frame "Data: Reorder Macro" {
        n147 = property on="Macro Steps" class="MCListbox (strict)"() -> ("ItemNames"=w319:string[][])  [unwired: 2 in, 2 out]
        n148 = Index Array(array=w319, index (col)=0 ("disabled index (col)")) -> (element=w317:string[])  [unwired: 1 in]
        n149 = Decimal String To Number(string=w317) -> (number=w316:i32[])  [unwired: 2 in, 1 out]
        n150 = Decrement(x=w316) -> (x-1=w313:i32[])
        n151 = in-place {
          in-place-border: w313 -> [w321]
          n152 = in-place-cluster #8(w315) -> ("Macro.New"=w323:refnum<class "Macro.lvclass">)
          n153 = call-dynamic "Reorder Steps.vi"("New Order"=w321, "Macro in"=w323) -> ("Macro out"=w322:refnum<class "Macro.lvclass">)  [unwired: 8 in, 1 out]
          n154 = in-place-cluster #8("Macro.New"=w322) -> (w314:T5)
        }
      }
      frame "Data: Save Macro" {
        n155 = Unbundle By Name(w327) -> ("Macro.New"=w324:refnum<class "Macro.lvclass">)
        n156 = call-dynamic "Write to File.vi"("error in (no error)"=w329, "Macro in"=w324) -> ("error out"=w328:errorcluster, "Macro out"=w325:refnum<class "Macro.lvclass">)  [unwired: 8 in]
        n157 = Bundle By Name(cluster=w327, "Macro.New"=w325, "Macro.Saved"=w325) -> (w326:T5)
      }
      frame "Data: Read Macro" {
        n158 = Unbundle By Name(w333) -> ("Macro Names"=w330:string[], "App Data Dir"=w331:path)
        n159 = in-place {
          in-place-border: w336 -> [w348]
          in-place-border: [w347] -> w335
          in-place-border: w331 -> [w343]
          in-place-border: w330 -> [w341]
          n160 = in-place-cluster #9(w333) -> ("Macro.New"=w346:refnum<class "Macro.lvclass">)  [unwired: 1 out]
          n161 = property class="Macro.lvclass"(reference=w346) -> (reference out=w342:refnum<class "Macro.lvclass">, "Accessors:Name"=w339:string)  [unwired: 1 in, 1 out]
          n162 = Search 1D Array(1D array=w341, element=w339) -> (index of element=w340:i32)  [unwired: 1 in]
          n163 = case shown="0, Default" w340 {
            tunnel: w348 -> [w354 w357]
            tunnel: [w353 w357] -> w347
            tunnel: w339 -> [w349 _]
            tunnel: w342 -> [_ w356]
            tunnel: [w352 _] -> w345
            tunnel: [w352 w355] -> w344
            tunnel: w343 -> [w351 _]
            frame 0, Default {
              n164 = call "Build Path to Macro.vi"("Macro Name"=w349, "App Data Dir"=w351) -> ("Macro File Path"=w350:path)  [unwired: 9 in]
              n165 = call "Load Macro from File.vi"("error in (no error)"=w354, "Path"=w350) -> ("error out"=w353:errorcluster, "Macro"=w352:refnum<class "Macro.lvclass">)  [unwired: 8 in]
            }
            frame -1 {
              n166 = call-dynamic "Clear Metadata.vi"("Macro in"=w356) -> ("Macro out"=w355:refnum<class "Macro.lvclass">)  [unwired: 9 in, 1 out]
            }
          }
          n167 = in-place-cluster #9("Macro.New"=w344, "Macro.Saved"=w345) -> (w334:T5)
        }
        n168 = property on="Macro Steps" class="MCListbox (strict)"("TopLeft"=T10 {"Row"=0, "Column"=0} ("Index Values")) -> ()  [unwired: 2 in, 2 out]
        n169 = call "Enqueue Multiple States.vi"("queue in"=w337, "State(s) at Back"="UI: Display Macro" ("State(s) at Back (\"\")")) -> ()  [unwired: 13 in, 1 out]
      }
      frame "Data: Flush Queue" {
        n170 = Flush Queue(queue=w358) -> ()  [unwired: 1 in, 3 out]
      }
      frame "Data: Cleanup" {
        # "Cleanup any data and references, here.\n(this is called automatically, by the Macro: Exit)"
        n171 = Unbundle By Name(w367) -> ("Core.Current VI Reference"=w366:refnum<vi>, "Keyboard"=w361:refnum<k1>)
        n172 = Close Reference(reference=w366, error in (no error)=w364) -> (error out=w362:errorcluster)
        n173 = call-poly <vilib>:"Close Input Device.vi"("error in (no error)"=w362, "device ID"=w361) -> ("error out"=w363:errorcluster)  [unwired: 8 in]
        n174 = invoke class="VI" method="Default Vals.Reinit All"(error in=w363) -> (error out=w365:errorcluster)  [unwired: 2 in, 2 out]
      }
      frame "---------- UI ----------" {
        # "Do not put any code in this frame.\n(It is a separator no-op. You can make a copy of this frame to create a new UI frame)"
      }
      frame "UI: Initialize" {
        # "Initialize the User Interface, here.\n(this is called automatically, by the Macro: Init)"
        n175 = property class="App"() -> ("Disp.AllMonitors"=w373:T16)  [unwired: 2 in, 2 out]
        n176 = for {
          tunnel: w373 -> [w384] mode=indexing
          tunnel: [w383] -> w371 mode=indexing
          n177 = Unbundle By Name(w384) -> ("Bounds.Right"=w382:i16, "Bounds.Left"=w380:i16, "Bounds.Bottom"=w381:i16, "Bounds.Top"=w379:i16)
          n178 = Subtract(x=w382, y=w380) -> (x-y=w377:i16)
          n179 = Subtract(x=w381, y=w379) -> (x-y=w378:i16)
          n180 = Bundle(w377, w378) -> (w383:cluster{i16, i16})  [unwired: 1 in]
        }
        "Resolutions" <- w371
        n181 = Array Size(array=w373) -> (size(s)=→"n Monitors":i32)
        n182 = property on="Start/Stop" class="Bool (strict)"("DisabledEnum"=T11."Disabled and Grayed Out" ("Disabled")) -> ()  [unwired: 2 in, 2 out]
        n183 = Bundle By Name(cluster=w372, "Resolutions"=w371) -> (w370:T5)
      }
      frame "UI: Uninitialize" {
        # "Uninitialize the User Interface, here.\n(this is called automatically, by the Macro: Exit)"
        n184 = property on="Dbl Click" class="Clust"("Position"=T12 {"Left"=864, "Top"=88}) -> ()  [unwired: 2 in, 2 out]
        n185 = property on="Add Step 2" class="Bool"("Position"=T12 {"Left"=864, "Top"=36}) -> ()  [unwired: 2 in, 2 out]
        n186 = property on="Start/Stop" class="Bool (strict)"("DisabledEnum"=T11."Disabled and Grayed Out" ("Disabled")) -> ()  [unwired: 2 in, 2 out]
        n187 = property on="Macro Name" class="CmbBox"("Strings[]"=string[] [] ("Strings []")) -> ()  [unwired: 2 in, 2 out]
        n188 = property on="Macro Steps" class="MCListbox (strict)"("TopLeft"=T10 {"Row"=0, "Column"=0} ("Index Values")) -> ()  [unwired: 2 in, 2 out]
        n189 = property on="Macro Steps" class="MCListbox (strict)"("ItemNames"=string[][] [] ("Item Names")) -> ()  [unwired: 2 in, 2 out]
      }
      frame "UI: Cursor Set" {
        # "Argument"
        # "Set and Unset Cursor Busy.\n(Usage: \"UI: Cursor Set >> Busy|Idle\")"
        n190 = case shown="\"Idle\", Default" w393 {
          tunnel: w395 -> [w398 w400]
          tunnel: [w397 w399] -> w394
          frame "Idle", Default {
            n191 = call <vilib>:"Unset Busy.vi"("error in (no error)"=w398) -> ("error out"=w397:errorcluster)  [unwired: 10 in]
          }
          frame "Busy" {
            n192 = call <vilib>:"Set Busy.vi"("error in (no error)"=w400) -> ("error out"=w399:errorcluster)  [unwired: 9 in, 1 out]
          }
        }
      }
      frame "UI: Front Panel State" {
        # "Argument"
        # "Set Front Panel Open or Closed\n(Usage: \"UI: Front Panel State >> Open|Close\")"
        n193 = Unbundle By Name(w403) -> ("Core.Current VI Reference"=w402:refnum<vi>)
        n194 = case shown="\"Open\", \"Standard\", Default" w401 {
          tunnel: w405 -> [w411 w426 w437 w450 w463]
          tunnel: [w413 w427 w439 w452 w465] -> w404
          tunnel: w402 -> [w412 w424 w438 w451 w464]
          frame "Open", "Standard", Default {
            w406 = T3."Standard" ("State")
            n195 = property class="VI"(reference=w412, error in=w411) -> (reference out=w409:refnum<vi>, error out=w410:errorcluster, "FP.State"=w408:T3)
            n196 = Not Equal?(x=w408, y=w406) -> (x != y?=w407:bool)
            n197 = case shown="True" w407 {
              tunnel: [w417 w419] -> w413
              tunnel: w410 -> [w416 w419]
              tunnel: w409 -> [w415 _]
              tunnel: w406 -> [w414 _]
              frame True {
                n198 = invoke class="VI" method="FP.Open"(reference=w415, error in=w416, "Activate"=TRUE, "State"=w414) -> (error out=w417:errorcluster)  [unwired: 1 in, 4 out]
              }
              frame False {
              }
            }
          }
          frame "Close", "Closed" {
            n199 = property class="VI"(reference=w424, error in=w426) -> (reference out=w423:refnum<vi>, error out=w425:errorcluster, "FP.State"=w421:T3)
            n200 = Not Equal?(x=w421, y=T3."Closed" ("Front Panel Window:State")) -> (x != y?=w420:bool)
            n201 = case shown="True" w420 {
              tunnel: [w428 w431] -> w427
              tunnel: w425 -> [w428 w430]
              tunnel: w423 -> [_ w429]
              frame False {
              }
              frame True {
                n202 = invoke class="VI" method="FP.Close"(reference=w429, error in=w430) -> (error out=w431:errorcluster)  [unwired: 1 in, 2 out]
              }
            }
          }
          frame "Hidden", "Hide" {
            w432 = T3."Hidden" ("State")
            n203 = property class="VI"(reference=w438, error in=w437) -> (reference out=w435:refnum<vi>, error out=w436:errorcluster, "FP.State"=w434:T3)
            n204 = Not Equal?(x=w434, y=w432) -> (x != y?=w433:bool)
            n205 = case shown="True" w433 {
              tunnel: [w443 w444] -> w439
              tunnel: w436 -> [w442 w444]
              tunnel: w435 -> [w441 _]
              tunnel: w432 -> [w440 _]
              frame True {
                n206 = invoke class="VI" method="FP.Open"(reference=w441, error in=w442, "State"=w440) -> (error out=w443:errorcluster)  [unwired: 2 in, 4 out]
              }
              frame False {
              }
            }
          }
          frame "Minimize", "Minimized" {
            w445 = T3."Minimized" ("State")
            n207 = property class="VI"(reference=w451, error in=w450) -> (reference out=w448:refnum<vi>, error out=w449:errorcluster, "FP.State"=w447:T3)
            n208 = Not Equal?(x=w447, y=w445) -> (x != y?=w446:bool)
            n209 = case shown="True" w446 {
              tunnel: [w456 w457] -> w452
              tunnel: w449 -> [w455 w457]
              tunnel: w448 -> [w454 _]
              tunnel: w445 -> [w453 _]
              frame True {
                n210 = invoke class="VI" method="FP.Open"(reference=w454, error in=w455, "State"=w453) -> (error out=w456:errorcluster)  [unwired: 2 in, 4 out]
              }
              frame False {
              }
            }
          }
          frame "Maximize", "Maximized" {
            w458 = T3."Maximized" ("State")
            n211 = property class="VI"(reference=w464, error in=w463) -> (reference out=w461:refnum<vi>, error out=w462:errorcluster, "FP.State"=w460:T3)
            n212 = Not Equal?(x=w460, y=w458) -> (x != y?=w459:bool)
            n213 = case shown="True" w459 {
              tunnel: [w469 w470] -> w465
              tunnel: w462 -> [w468 w470]
              tunnel: w461 -> [w467 _]
              tunnel: w458 -> [w466 _]
              frame True {
                n214 = invoke class="VI" method="FP.Open"(reference=w467, error in=w468, "State"=w466) -> (error out=w469:errorcluster)  [unwired: 2 in, 4 out]
              }
              frame False {
              }
            }
          }
        }
      }
      frame "UI: Interlocks" {
        n215 = Unbundle By Name(w475) -> ("Refs"=w474:T7, "Macro.New"=w473:refnum<class "Macro.lvclass">, "Macro.Saved"=w472:refnum<class "Macro.lvclass">)
        n216 = Current VI's Menubar() -> (w471:refnum<k9>)
        n217 = call "UI Interlocks.vi"("Menu Ref"=w471, "Saved Macro"=w472, "New Macro"=w473, "Refs"=w474) -> ()  [unwired: 7 in, 1 out]
      }
      frame "UI: Process Menu Selection" {
        n218 = Current VI's Menubar() -> (w480:refnum<k9>)
        n219 = call "Process Menu Selection.vi"("error in (no error)"=w482, "Argument"=w479, "Menu Ref"=w480) -> ("error out"=w481:errorcluster, "State(s) to Enqueue"=w477:string)  [unwired: 7 in]
        n220 = call "Enqueue Multiple States.vi"("queue in"=w478, "State(s) at Back"=w477) -> ()  [unwired: 13 in, 1 out]
      }
      frame "UI: Populate Macros" {
        n221 = Unbundle By Name(w487) -> ("App Data Dir"=w485:path)
        n222 = call "Read Macro Names.vi"("error in (no error)"=w490, "App Data Directory"=w485) -> ("error out"=w489:errorcluster, "Macro Names"=w486:string[])  [unwired: 8 in]
        n223 = Sort 1D Array(array=w486) -> (sorted array=w484:string[])
        n224 = Bundle By Name(cluster=w487, "Macro Names"=w484) -> (w488:T5)
        n225 = property on="Macro Name" class="CmbBox"("Strings[]"=w484) -> ()  [unwired: 2 in, 2 out]
      }
      frame "UI: Display Macro" {
        n226 = Unbundle By Name(w499) -> ("Macro.New"=w498:refnum<class "Macro.lvclass">)
        n227 = property class="Macro.lvclass"(reference=w498) -> (reference out=w494:refnum<class "Macro.lvclass">, "Accessors:Description"=w491:string, "Accessors:Activation Type"=w492:enum32{"Hotkey", "Automatic"}, "Accessors:N"=w493:i32)  [unwired: 1 in, 1 out]
        n228 = call-dynamic "Display Data.vi"("Macro in"=w494) -> ("Metadata"=→"Metadata":string, "Macro Steps"=w495:string[][])  [unwired: 7 in, 2 out]
        n229 = local write "Description"(w491) -> ()
        n230 = local write "Activation Type"(w492) -> ()
        n231 = local write "N"(w493) -> ()
        n232 = property on="Macro Steps" class="MCListbox (strict)"("ItemNames"=w495) -> ()  [unwired: 2 in, 2 out]
      }
      frame "UI: Update Status" {
        n233 = case shown="\"Restore\"" w501 {
          tunnel: w502 -> [_ _ w512 w518 w524 w530 w536 _ _]
          tunnel: ["Idle" "Listening for hotkey press" w508 w513 w519 w525 w531 "Macro saved" ("Status") "Macro restored to last save" ("Status")] -> w500
          frame "Idle", Default {
          }
          frame "Listen" {
          }
          frame "Step" {
            n234 = Unbundle By Name(w512) -> ("n"=w506:i32, "Rcount"=w507:i32, "Macro.New"=w511:refnum<class "Macro.lvclass">, "Step"=w510:i32, "Start Time"=w509:timestamp)
            n235 = call-dynamic "Build Status Message.vi"("Macro Repeat"=w506, "Step Repeat"=w507, "Start Time"=w509, "Step"=w510, "Macro in"=w511) -> ("Status"=w508:string)  [unwired: 4 in, 2 out]
          }
          frame "Complete Idle" {
            n236 = Unbundle By Name(w518) -> ("Start Time"=w516:timestamp)
            n237 = Get Date/Time In Seconds() -> (seconds since 1Jan1904=w515:timestamp)
            n238 = Subtract(x=w515, y=w516) -> (x-y=w514:dbl)
            n239 = Format Into String(format string="Macro completed in %.3t s.\nIdle", w514) -> (resulting string=w513:string)  [unwired: 2 in, 1 out]
          }
          frame "Complete Listen" {
            n240 = Unbundle By Name(w524) -> ("Start Time"=w522:timestamp)
            n241 = Get Date/Time In Seconds() -> (seconds since 1Jan1904=w521:timestamp)
            n242 = Subtract(x=w521, y=w522) -> (x-y=w520:dbl)
            n243 = Format Into String(format string="Macro completed in %.3t s.\nListening for hotkey press", w520) -> (resulting string=w519:string)  [unwired: 2 in, 1 out]
          }
          frame "Abort Idle" {
            n244 = Unbundle By Name(w530) -> ("Start Time"=w528:timestamp)
            n245 = Get Date/Time In Seconds() -> (seconds since 1Jan1904=w527:timestamp)
            n246 = Subtract(x=w527, y=w528) -> (x-y=w526:dbl)
            n247 = Format Into String(format string="Macro aborted after %.3t s.\nIdle", w526) -> (resulting string=w525:string)  [unwired: 2 in, 1 out]
          }
          frame "Abort Listen" {
            n248 = Unbundle By Name(w536) -> ("Start Time"=w534:timestamp)
            n249 = Get Date/Time In Seconds() -> (seconds since 1Jan1904=w533:timestamp)
            n250 = Subtract(x=w533, y=w534) -> (x-y=w532:dbl)
            n251 = Format Into String(format string="Macro aborted after %.3t s.\nListening for hotkey press", w532) -> (resulting string=w531:string)  [unwired: 2 in, 1 out]
          }
          frame "Save" {
          }
          frame "Restore" {
          }
        }
        "Status" <- w500
      }
      frame "UI: Wait" {
        n252 = Unbundle By Name(w546) -> ("Keyboard"=w544:refnum<k1>, "Hotkey Values"=w543:T6)
        n253 = call "Check for Hotkey Press.vi"("Hotkey Type"=Hotkey_Type."Abort Hotkey", "error in (no error)"=w549, "Hotkeys"=w543, "Keyboard"=w544) -> ("error out"=w545:errorcluster, "Pressed?"=w541:bool)  [unwired: 5 in, 1 out]
        n254 = call "Timer FGV.vi"("Mode"=FGV_Actions."Read", "error in (no error)"=w545) -> ("error out"=w552:errorcluster, "Expired?"=w550:bool)  [unwired: 7 in, 1 out]
        n255 = case "Abort pressed?" shown="False" w541 {
          tunnel: w550 -> [w556 _]
          tunnel: [w553 "Macro: Process >> Abort" ("t")] -> w548
          frame False {
            n256 = Select(t="Macro: Process >> Count", s=w556, f="UI: Wait") -> (s? t:f=w553:string)
          }
          frame True {
          }
        }
        n257 = call "Stall Data Flow.vim"("value in"=w552, "milliseconds to wait"=u32 1) -> ("value out"=w540:errorcluster)  [unwired: 1 out]
        n258 = call "Enqueue Multiple States.vi"("queue in"=w547, "State(s) at Back"=w548) -> ()  [unwired: 13 in, 1 out]
      }
      frame "UI: Listen" {
        n259 = Unbundle By Name(w565) -> ("Keyboard"=w570:refnum<k1>, "Hotkey Values"=w560:T6)
        n260 = call "Stall Data Flow.vim"("value in"=w570, "milliseconds to wait"=u32 1) -> ("value out"=w568:refnum<k1>)  [unwired: 1 out]
        n261 = call "Check for Hotkey Press.vi"("Hotkey Type"=Hotkey_Type."Macro Hotkey", "error in (no error)"=w566, "Hotkeys"=w560, "Keyboard"=w568) -> ("error out"=w561:errorcluster, "Pressed?"=w558:bool)  [unwired: 5 in, 1 out]
        n262 = Select(t="Macro: Process >> Proc", s=w558, f="UI: Listen" ("string")) -> (s? t:f=w564:string)
        n263 = call "Enqueue Multiple States.vi"("queue in"=w562, "State(s) at Back"=w564) -> ()  [unwired: 13 in, 1 out]
      }
      frame "UI: Settings" {
        n264 = call "Change Settings.vi"("error in (no error)"=w572) -> ("error out"=w571:errorcluster)  [unwired: 10 in]
      }
      frame "UI: Help" {
        n265 = call "Display Help Message to User"("error in (no error)"=w575) -> ("error out"=w574:errorcluster)  [unwired: 9 in, 1 out]
      }
      frame "UI: Prompt for Save" {
        n266 = Unbundle By Name(w582) -> ("Macro.New"=w579:refnum<class "Macro.lvclass">)
        n267 = property class="Macro.lvclass"(reference=w579) -> ("Accessors:Path"=w578:path)  [unwired: 1 in, 2 out]
        n268 = Empty String/Path?(string/path=w578) -> (empty?=w577:bool)
        n269 = case shown="True" w577 {
          tunnel: ["UI: Save As" w586] -> w581
          frame True {
          }
          frame False {
            n270 = call "Overwrite?"() -> ("OK"=w585:bool)  [unwired: 10 in, 1 out]
            n271 = Select(t="Macro: Save Macro", s=w585, f="") -> (s? t:f=w586:string)
          }
        }
        n272 = call "Enqueue Multiple States.vi"("queue in"=w583, "State(s) at Back"=w581) -> ()  [unwired: 13 in, 1 out]
      }
      frame "UI: Save As" {
        n273 = in-place {
          in-place-border: [w594] -> w590
          n274 = in-place-cluster #10(w593) -> ("Macro.New"=w602:refnum<class "Macro.lvclass">)
          n275 = property class="Macro.lvclass"(reference=w602) -> (reference out=w599:refnum<class "Macro.lvclass">, "Accessors:Name"=w603:string)  [unwired: 1 in, 1 out]
          n276 = call "File Dialog2"("prompt"="Save As", "default name"=w603, "pattern (all files)"="*.ini", "pattern label"="Configuration Files") -> ("selected path"=w601:path, "cancelled"=w597:bool, "error out"=w607:errorcluster)  [unwired: 8 in, 1 out]
          n277 = property class="Macro.lvclass"(reference=w599, "Accessors:Path"=w601) -> (reference out=w600:refnum<class "Macro.lvclass">)  [unwired: 1 in, 1 out]
          n278 = call <vilib>:"Clear Errors.vi"("error in (no error)"=w607) -> ()  [unwired: 5 in, 2 out]
          n279 = Select(t="", s=w597, f="Macro: Save Macro") -> (s? t:f=w594:string)
          n280 = Select(t=w599, s=w597, f=w600) -> (s? t:f=w598:refnum<class "Macro.lvclass">)
          n281 = in-place-cluster #10("Macro.New"=w598) -> (w591:T5)
        }
        n282 = call "Enqueue Multiple States.vi"("queue in"=w592, "State(s) at Back"=w590) -> ()  [unwired: 13 in, 1 out]
      }
      frame "UI: Confirm Exit" {
        n283 = Unbundle By Name(w616) -> ("Macro.New"=w612:refnum<class "Macro.lvclass">, "Macro.Saved"=w613:refnum<class "Macro.lvclass">)
        n284 = Not Equal?(x=w612, y=w613) -> (x != y?=w611:bool)
        n285 = call "Exit anyway?"("Enable"=w611) -> ("Exit"=w615:bool)  [unwired: 9 in, 1 out]
        n286 = Implies(1:w615, 2:w611) -> (0:w609:bool)
        n287 = case shown="True" w609 {
          tunnel: w614 -> [w617 w621]
          tunnel: [w617 w620] -> w610
          tunnel: w608 -> [_ w619]
          frame False {
          }
          frame True {
            n288 = Generate User Event(user event=w619, event data cluster=TRUE ("event data"), error in=w621) -> (error out=w620:errorcluster)  [unwired: 1 in, 1 out]
          }
        }
      }
      frame "---------- Macro ----------" {
        # "Do not put any code in this frame.\n(It is a separator no-op. You can make a copy of this frame to create a new Macro frame)"
      }
      frame "Macro: Initialize" {
        w624 = "Data: Initialize\nData: Bundle Refs\nInitialize Core Data\nUI: Initialize\nData: Get Hotkey\nUI: Populate Macros\nUI: Interlocks\nUI: Front Panel State >> Open\nUI: Update Status >> Idle"  # Data: Initialize Data: Bundle Refs Initialize Core Data UI: Initialize Data: Get Hotkey UI: Populate Macros UI: Interlocks UI: Front Panel State >> Open UI: Update Status >> Idle
        # "Initialization Macro\n(This is called once, when the VI starts)"
        n289 = call "Enqueue Multiple States.vi"("State(s) at Front"=w624, "queue in"=w627) -> ()  [unwired: 13 in, 1 out]
      }
      frame "Macro: Save Macro" {
        n290 = call "Enqueue Multiple States.vi"("State(s) at Front"="Data: Bundle Macro\nData: Save Macro\nUI: Populate Macros\nUI: Update Status >> Save\nUI: Interlocks", "queue in"=w631) -> ()  [unwired: 13 in, 1 out]
      }
      frame "Macro: Process" {
        n291 = case shown="\"Count\"" w636 {
          tunnel: w633 -> [w639 w648 w658 w671 w684 w690 w693 w700]
          tunnel: [w639 w651 w657 w669 w682 w689 w693 w700] -> w635
          tunnel: [w641 "UI: Interlocks\nMacro: Process >> Step" w655 w667 w680 "UI: Update Status >> Step\nProcess: Perform Step" w694 w701] -> w634
          frame "Start", Default {
            # "Reached when Start button is pressed"
            n292 = Unbundle By Name(w639) -> ("Macro.New"=w640:refnum<class "Macro.lvclass">)
            n293 = property class="Macro.lvclass"(reference=w640) -> ("Accessors:Activation Type"=w638:enum32{"Hotkey", "Automatic"})  [unwired: 1 in, 2 out]
            n294 = Equal?(x=w638, y=enum32{"Hotkey", "Automatic"}."Hotkey") -> (x = y?=w645:bool)
            n295 = Select(t="UI: Interlocks\nUI: Update Status >> Listen\nUI: Listen", s=w645, f="Macro: Proc") -> (s? t:f=w641:string)
          }
          frame "Proc" {
            w650 = 0 ("Step")
            # "Reached when Macro hotkey is activated or right after Start button for Automatic activation type"
            n296 = Get Date/Time In Seconds() -> (seconds since 1Jan1904=w649:timestamp)
            n297 = Bundle By Name(cluster=w648, "Step"=w650, "n"=w650, "Rcount"=w650, "Start Time"=w649, "Report Data"=T8[] []) -> (w651:T5)
          }
          frame "Step" {
            # "Reached when a macro procs, or the current step of a macro finishes executing"
            n298 = Unbundle By Name(w658) -> ("Step"=w661:i32, "Macro.New"=w653:refnum<class "Macro.lvclass">)
            n299 = call-dynamic "Get Step Count.vi"("Macro in"=w653) -> ("Step Count"=w652:i32)  [unwired: 8 in, 2 out]
            n300 = Less?(x=w661, y=w652) -> (x < y?=w660:bool)
            n301 = Bundle By Name(cluster=w658, "Step"=w661, "Rcount"=0) -> (w657:T5)
            n302 = Select(t="UI: Update Status >> Step\nProcess: Perform Step\nUI: Wait", s=w660, f="Macro: Process >> End") -> (s? t:f=w655:string)
          }
          frame "Count" {
            # "Reached when one count of the current step of a macro finishes executing"
            n303 = Unbundle By Name(w671) -> ("Rcount"=w666:i32, "Macro.New"=w665:refnum<class "Macro.lvclass">, "Step"=w664:i32)
            n304 = call-dynamic "Index Steps.vi"("Index"=w664, "Macro in"=w665) -> ("Step"=w663:refnum<class "Step.lvclass">)  [unwired: 7 in, 2 out]
            n305 = property class="Step.lvclass"(reference=w663) -> ("Accessors:Repeat"=w662:i32)  [unwired: 1 in, 2 out]
            n306 = Increment(x=w666) -> (x+1=w670:i32)
            n307 = Greater Or Equal?(x=w666, y=w662) -> (x >= y?=w673:bool)
            n308 = Bundle By Name(cluster=w671, "Rcount"=w670) -> (w669:T5)
            n309 = Select(t="Data: Increment Step\nMacro: Process >> Step", s=w673, f="UI: Update Status >> Step\nProcess: Perform Step\nUI: Wait") -> (s? t:f=w667:string)
          }
          frame "End" {
            # "Reached when the last step of a macro finishes executing"
            n310 = Unbundle By Name(w684) -> ("n"=w686:i32, "Macro.New"=w675:refnum<class "Macro.lvclass">)
            n311 = property class="Macro.lvclass"(reference=w675) -> ("Accessors:N"=w674:i32)  [unwired: 1 in, 2 out]
            n312 = Increment(x=w686) -> (x+1=w683:i32)
            n313 = Greater?(x=w683, y=w674) -> (0:w678:bool)
            n314 = Not Equal?(x=w674, y=-1) -> (x != y?=w677:bool)
            n315 = And(x=w678, y=w677) -> (x .and. y?=w676:bool)
            n316 = Bundle By Name(cluster=w684, "n"=w683) -> (w682:T5)
            n317 = Select(t="Macro: Process >> Complete", s=w676, f="Macro: Process >> Repeat") -> (s? t:f=w680:string)
          }
          frame "Repeat" {
            w687 = 0 ("Step")
            # "Reached when a whole macro needs to be repeated"
            n318 = Bundle By Name(cluster=w690, "Step"=w687, "Rcount"=w687) -> (w689:T5)
          }
          frame "Complete" {
            # "Reached when a macro fully finishes including all repeats"
            n319 = Unbundle By Name(w693) -> ("Macro.New"=w692:refnum<class "Macro.lvclass">)
            n320 = property class="Macro.lvclass"(reference=w692) -> ("Accessors:Activation Type"=w691:enum32{"Hotkey", "Automatic"})  [unwired: 1 in, 2 out]
            n321 = case shown="\"Automatic\"" w691 {
              tunnel: ["Data: Build Report\nUI: Update Status >> Complete Listen\nUI: Listen" "UI: Update Status >> Complete Idle"] -> w694
              frame "Hotkey" {
              }
              frame "Automatic" {
                n322 = property on="Start/Stop" class="Bool (strict)"("Val(Sgnl)"=FALSE ("Value (Signaling)")) -> ()  [unwired: 2 in, 2 out]
              }
            }
          }
          frame "Abort" {
            # "Reached when Abort hotkey is detected"
            n323 = Unbundle By Name(w700) -> ("Macro.New"=w699:refnum<class "Macro.lvclass">)
            n324 = property class="Macro.lvclass"(reference=w699) -> ("Accessors:Activation Type"=w698:enum32{"Hotkey", "Automatic"})  [unwired: 1 in, 2 out]
            n325 = case shown="\"Automatic\"" w698 {
              tunnel: ["UI: Update Status >> Abort Listen\nUI: Listen" "UI: Update Status >> Abort Idle"] -> w701
              frame "Hotkey" {
              }
              frame "Automatic" {
                n326 = property on="Start/Stop" class="Bool (strict)"("Val(Sgnl)"=FALSE ("Value (Signaling)")) -> ()  [unwired: 2 in, 2 out]
              }
            }
          }
        }
        n327 = call "Enqueue Multiple States.vi"("queue in"=w632, "State(s) at Back"=w634) -> ()  [unwired: 13 in, 1 out]
      }
      frame "Macro: Exit" {
        # "Exit Macro\n(This is called once, when the VI exits)"
        n328 = Unbundle By Name(w713) -> ("Core.Close Panel on Exit?"=w712:bool)
        n329 = Select(t="\nUI: Front Panel State >> Close", s=w712, f="") -> (s? t:f=w708:string)
        n330 = Concatenate Strings("UI: Uninitialize\n", w708, "Data: Cleanup\nExit") -> (w707:string)
        n331 = call "Enqueue Multiple States.vi"("State(s) at Front"=w707, "queue in"=w709) -> ()  [unwired: 13 in, 1 out]
      }
      frame "---------- Process ----------" {
      }
      frame "Process: Perform Step" {
        n332 = Unbundle By Name(w724) -> ("Macro.New"=w719:refnum<class "Macro.lvclass">, "Step"=w718:i32)
        n333 = call-dynamic "Index Steps.vi"("Index"=w718, "Macro in"=w719) -> ("Step"=w717:refnum<class "Step.lvclass">)  [unwired: 7 in, 2 out]
        n334 = call-dynamic "Perform Step.vi"("error in (no error)"=w722, "Step in"=w717) -> ("error out"=w721:errorcluster, "Result"=w720:T8)  [unwired: 7 in, 1 out]
        n335 = in-place {
          in-place-border: w720 -> [w726]
          n336 = in-place-cluster #11(w724) -> ("Report Data"=w728:T8[])
          n337 = Build Array (concatenate)(w728, w726) -> (w727:T8[])
          n338 = in-place-cluster #11("Report Data"=w727) -> (w723:T5)
        }
        n339 = call "Enqueue Multiple States.vi"("queue in"=w725) -> ()  [unwired: 14 in, 1 out]
      }
    }
  }
  n340 = Merge Errors(w8, w7) -> (w9:errorcluster)
  n341 = Release Queue(queue=w10, error in (no error)=w9) -> (error out=→"error out":errorcluster)  [unwired: 1 in, 2 out]
